vi "CodifyFrequency(Single).vi"(1 "Frequency In":dbl=60.0 min=60.0 max=90.0 step=0.1) -> (0 "32bit integer":u32)   [LabVIEW 2017, in "AODControl.lvlib"]
uses:
  AODControl.lvlib
panel:
  out "Boolean array":bool[](array[boolean])
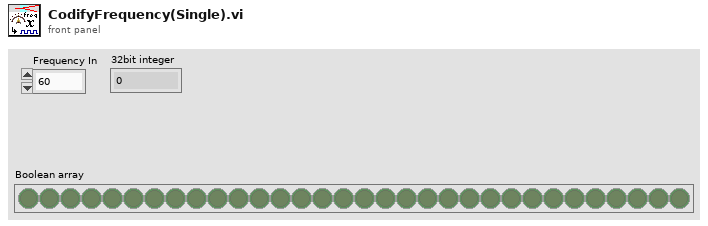
[diagram p1: front panel]
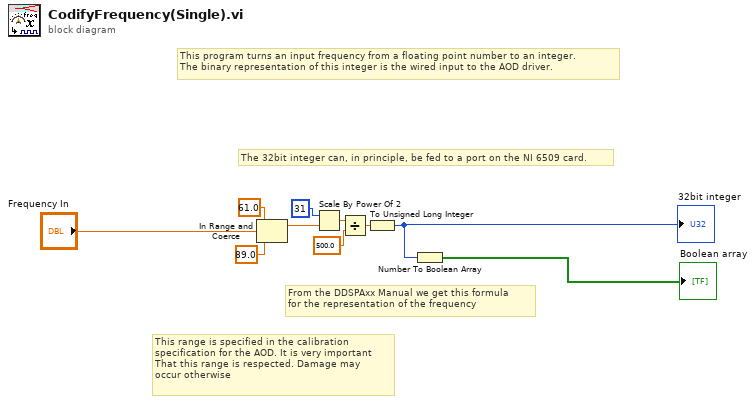
[diagram p0: block diagram]
diagram:
  # "The 32bit integer can, in principle, be fed to a port on the NI 6509 card."
  # "From the DDSPAxx Manual we get this formula\nfor the representation of the frequency"
  # "This range is specified in the calibration\nspecification for the AOD. It is very important\nThat this range is respected. Damage may \noccur otherwise"
  # "This program turns an input frequency from a floating point number to an integer. \nThe binary representation of this integer is the wired input to the AOD driver."
  n1 = In Range and Coerce(upper limit=61.0, x="Frequency In", lower limit=89.0) -> (coerced(x)=w3:dbl)  [unwired: 1 out]
  n2 = Scale By Power Of 2(n=i16 31, x=w3) -> (x*2^n=w9:dbl)
  n3 = Divide(x=w9, y=500.0) -> (x/y=w6:dbl)
  n4 = To Unsigned Long Integer(number=w6) -> (unsigned 32bit integer=w5:u32)
  "32bit integer" <- w5
  n5 = Number To Boolean Array(number=w5) -> (Boolean array=→"Boolean array":bool[])
